vi "Read configuration.vi"(8 "error in":errorcluster, 11 "Cfg Channel in":refnum<class "channel node.lvclass">) -> (0 "error out":errorcluster, 2 "configuration":refnum<class "NISE_CEF_serializable configuration.lvclass">, 3 "Cfg Channel out":refnum<class "channel node.lvclass">)   [LabVIEW 2013, in "channel node.lvclass"]
uses:
  channel node.lvclass
  Configuration Framework/serializable configuration/NISE_CEF_serializable configuration.lvclass
  channel node.lvclass/channel node.ctl
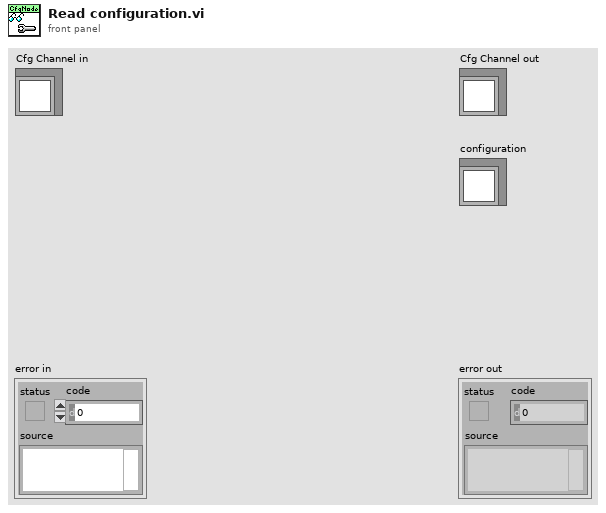
[diagram p1: front panel]
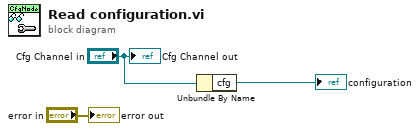
[diagram p0: block diagram]
diagram:
  n1 = Unbundle By Name("Cfg Channel in") -> ("cfg"=→"configuration":refnum<class "channel configuration.lvclass">)
  "error out" <- "error in"
  "Cfg Channel out" <- "Cfg Channel in"
